vi "initialize AO task.vi"(7 "rate":dbl=1000.0 format="%0.2f", 8 "error in":errorcluster, 10 "waveform":dbl[][](array[numeric]) format="%0.2f", 11 "AO Connection":T1) -> (0 "error out":errorcluster, 3 "task out":refnum<k21>)   [LabVIEW 2021, in "NI.lvlib" / "NI.lvclass"]
uses:
  NI.lvclass
  Channel Connection.ctl
  <vilib>/DAQmx/write.llb/DAQmx Write (Analog 2D DBL NChan NSamp).vi
  <vilib>/DAQmx/create/channels.llb/DAQmx Create Channel (AO-Voltage-Basic).vi
  <vilib>/DAQmx/configure/timing.llb/DAQmx Timing (Sample Clock).vi
  <vilib>/DAQmx/configure/trigger.llb/DAQmx Start Trigger (Digital Edge).vi
  <vilib>/DAQmx/miscellaneous.llb/DAQmx Fill In Error Info.vi
  <resource>/objmgr/daqmx.rc
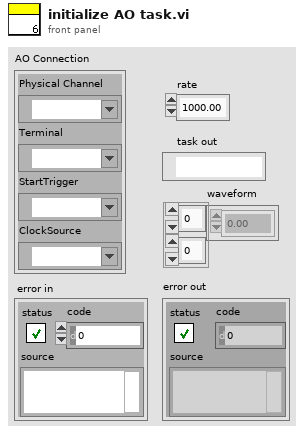
[diagram p1: front panel]
types:
  T1 = typedef "NI.lvlib/NI.lvclass/Channel Connection.ctl" = cluster{"Physical Channel":tag, "Terminal":tag, "StartTrigger":tag, "ClockSource":tag}
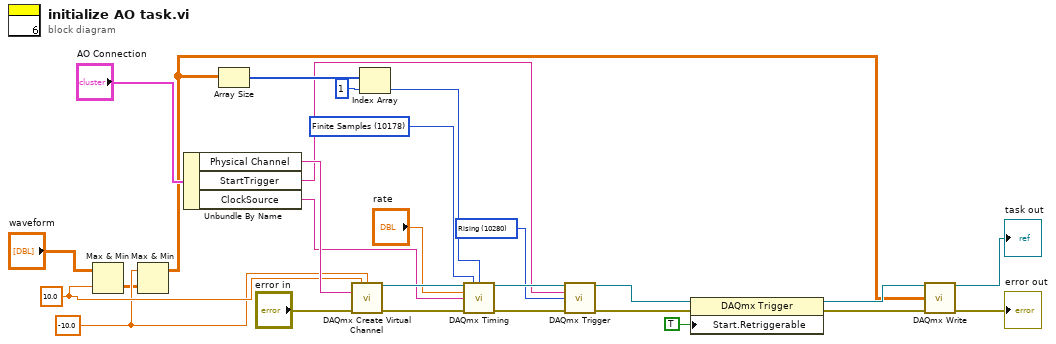
[diagram p0: block diagram]
diagram:
  w3 = -10.0 ("minimum value")
  w5 = 10.0 ("maximum value")
  w12 = 10280 items=["Rising"=10280, "Falling"=10171] ("edge")
  w27 = 10178 items=["Finite Samples"=10178, "Continuous Samples"=10123, "Hardware Timed Single Point"=12522] ("sample mode")
  n1 = Max & Min(x="waveform", y=w5) -> (min(x,y)=w2:dbl[][])  [unwired: 1 out]
  n2 = Max & Min(x=w3, y=w2) -> (max(x,y)=w1:dbl[][])  [unwired: 1 out]
  n3 = Unbundle By Name("AO Connection") -> ("Physical Channel"=w19:tag, "StartTrigger"=w13:tag, "ClockSource"=w14:tag)
  n4 = Array Size(array=w1) -> (size(s)=w18:i32[])
  n5 = call-poly <vilib>:"DAQmx Create Virtual Channel.vi"("maximum value"=w5, "minimum value"=w3, "physical channels"=w19, "error in"="error in") -> ("task out"=w25:refnum<k21>, "error out"=w26:errorcluster)  [unwired: 10 in]
  n6 = Index Array(array=w18, index=1) -> (element=w16:i32)
  n7 = call-poly <vilib>:"DAQmx Timing.vi"("task/channels in"=w25, "sample mode"=w27, "samples per channel"=w16, "rate"="rate", "source"=w14, "error in"=w26) -> ("task out"=w22:refnum<k21>, "error out"=w23:errorcluster)  [unwired: 8 in]
  n8 = call-poly <vilib>:"DAQmx Trigger.vi"("task/channels in"=w22, "source"=w13, "edge"=w12, "error in"=w23) -> ("task out"=w24:refnum<k21>, "error out"=w8:errorcluster)  [unwired: 10 in]
  n9 = property class="DAQmx Trigger"(reference=w24, error in=w8, "Start.Retriggerable"=TRUE) -> (reference out=w21:refnum<k21>, error out=w6:errorcluster)
  n10 = call-poly <vilib>:"DAQmx Write.vi"("task/channels in"=w21, "data"=w1, "error in"=w6) -> ("task out"=→"task out":refnum<k21>, "error out"=→"error out":errorcluster)  [unwired: 10 in, 1 out]
